vi "CreateListImp.vi"(8 "error in (no error)":errorcluster, 11 "List in":refnum<class "ObjectList.lvclass">) -> (0 "error out":errorcluster, 3 "List out":refnum<class "ObjectList.lvclass">)   [LabVIEW 2013, in "LapDog.Collections.v_.Lists.lvlib" / "ObjectList.lvclass"]
uses:
  ObjectList.lvclass
  ListImp/ListImp.lvclass
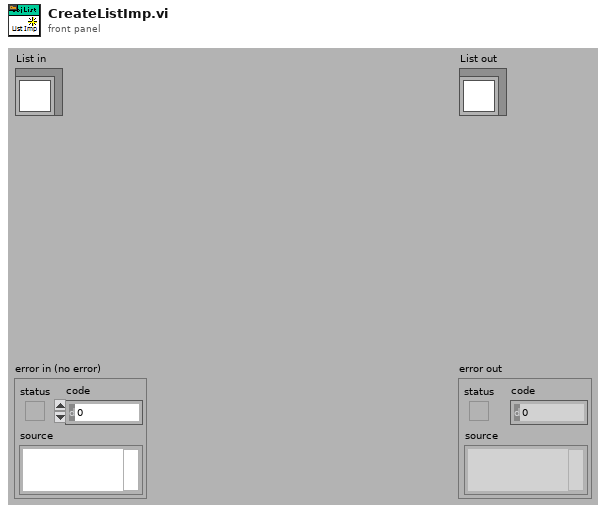
[diagram p1: front panel]
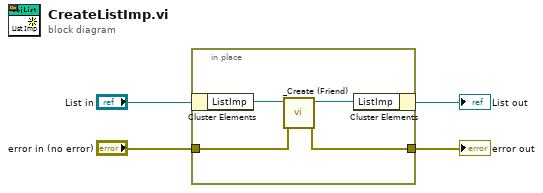
[diagram p0: block diagram]
diagram:
  n1 = in-place {
    in-place-border: "error in (no error)" -> [w6]
    in-place-border: [w5] -> w1
    n2 = in-place-cluster #1("List in") -> ("ListImp"=w8:refnum<class "ListImp.lvclass">)
    n3 = call "_Create (Friend).vi"("error in (no error)"=w6, "ListImp in"=w8) -> ("error out"=w5:errorcluster, "ListImp out"=w7:refnum<class "ListImp.lvclass">)  [unwired: 8 in]
    n4 = in-place-cluster #1("ListImp"=w7) -> (→"List out":refnum<class "ObjectList.lvclass">)
  }
  "error out" <- w1
